vi "dtCalculatorandArrayIntegration.vi"(11 "Data Input":dbl[][](array[numeric])) -> (3 "output array":dbl[][](array[numeric]))   [LabVIEW 2026]
panel:
  out "Timing Array Out":dbl[](array[numeric])
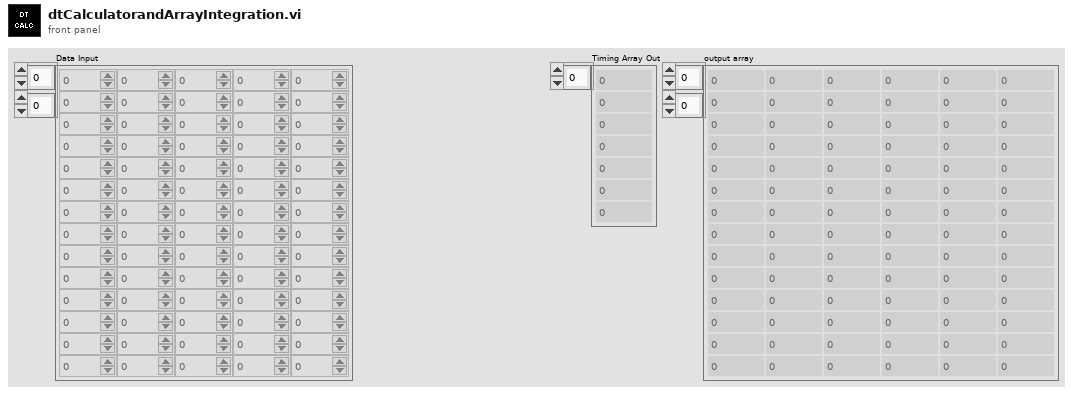
[diagram p1: front panel]
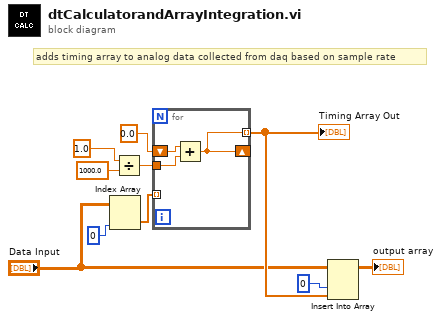
[diagram p0: block diagram]
diagram:
  # "adds timing array to analog data collected from daq based on sample rate"
  n1 = Index Array(array="Data Input", index (col)=0 ("disabled index (col)")) -> (element=w10:dbl[])  [unwired: 1 in]
  n2 = Divide(x=1.0, y=1000.0) -> (x/y=w7:dbl)
  n3 = for {
    tunnel: w10 -> [_] mode=indexing
    tunnel: w7 -> [w13]
    shift-right: [w11] -> _
    shift-left: 0.0 -> [w12]
    tunnel: [w11] -> w4 mode=indexing
    n4 = Add(x=w12, y=w13) -> (x+y=w11:dbl)
  }
  "Timing Array Out" <- w4
  n5 = Insert Into Array(array="Data Input", index (col)=0 ("disabled index (col)"), new element=w4) -> (→"output array":dbl[][])  [unwired: 1 in]
